vi "Process Image.vi"(4 "Path Angle":dbl, 6 "Camera Angle":dbl, 7 "Upper Threshold":dbl, 8 "Error In":errorcluster, 9 "FOV":dbl[](array[numeric]), 10 "Process Memory":T1, 11 "Acquired Image":T1) -> (0 "Error Out":errorcluster, 1 "Particle Locations":dbl[][](array[numeric]) format="%.2f", 2 "Processed Image":T1)   [LabVIEW 2017]
uses:
  <vilib>/vision/Image Controls.llb/IMAQ Image.ctl
  <vilib>/vision/NI_Vision_Development_Module.lvlib
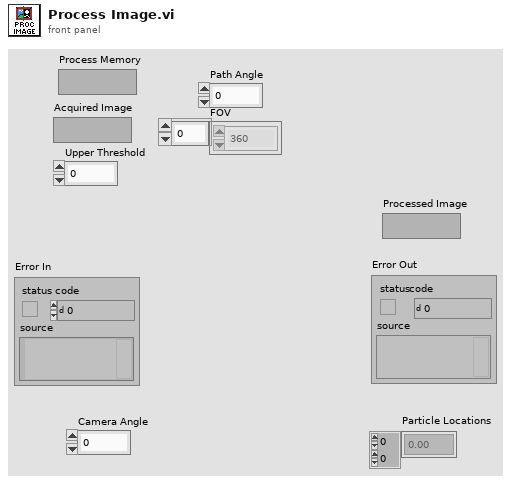
[diagram p1: front panel]
types:
  T1 = typedef "IMAQ Image.ctl" = refnum<image>
  T2 = typedef "IMAQ Circle" = cluster{"Center X":i32, "Center Y":i32, "Inner Radius":i32, "Outer Radius":i32, "Start Angle":dbl, "End Angle":dbl}
  T3 = typedef "Particle Parameters" = i32
  T4 = typedef "ROI Descriptor" = cluster{"Global Rectangle":i32[], "Contours":cluster{"ID":enum32{"External", "Internal"}, "Type":u32, "Coordinates":i32[]}[]}
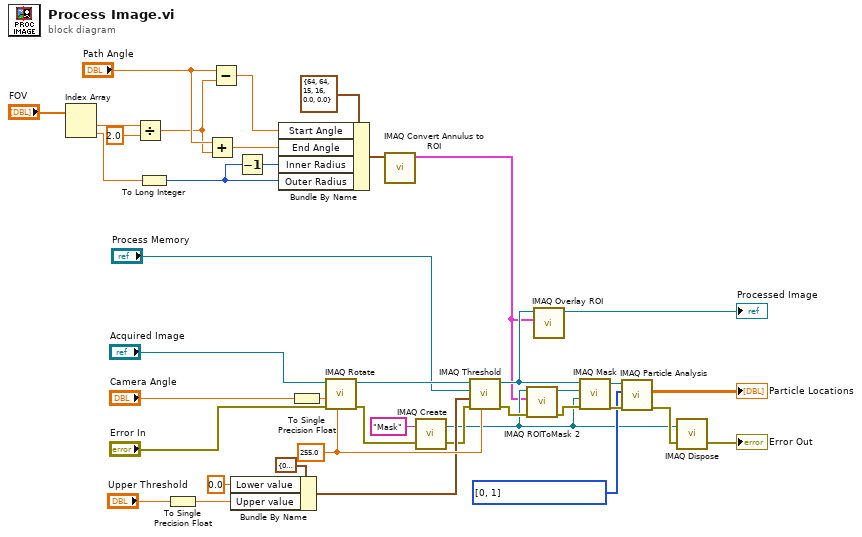
[diagram p0: block diagram]
diagram:
  w33 = T3[] [0, 1] items=["Center of Mass X", "Center of Mass Y", "First Pixel X", "First Pixel Y", "Bounding Rect Left", "Bounding Rect Top", "Bounding Rect Right", "Bounding Rect Bottom", "Max Feret Diameter Start X", "Max Feret Diameter Start Y", "Max Feret Diameter End X", "Max Feret Diameter End Y", "Max Horiz. Segment Length Left", "Max Horiz. Segment Length Right", "Max Horiz. Segment Length Row", "-", "Bounding Rect Width", "Bounding Rect Height", "Bounding Rect Diagonal", "Perimeter", "Convex Hull Perimeter", "Holes' Perimeter", "Max Feret Diameter", "Equivalent Ellipse Major Axis", "Equivalent Ellipse Minor Axis", "Equivalent Ellipse Minor Axis (Feret)", "Equivalent Rect Long Side", "Equivalent Rect Short Side", "Equivalent Rect Diagonal", "Equivalent Rect Short Side (Feret)", "Average Horiz. Segment Length", "Average Vert. Segment Length", "Hydraulic Radius", "Waddel Disk Diameter", "-", "Area", "Holes' Area", "Particle & Holes' Area", "Convex Hull Area", "Image Area", "-", "Number of Holes", "Number of Horiz. Segments", "Number of Vert. Segments", "-", "Orientation", "Max Feret Diameter Orientation", "-", "% Area/Image Area", "% Area/(Particle & Holes' Area)", "Ratio of Equivalent Ellipse Axes", "Ratio of Equivalent Rect Sides", "-", "Elongation Factor", "Compactness Factor", "Heywood Circularity Factor", "Type Factor", "-", "Sum X", "Sum Y", "Sum XX", "Sum XY", "Sum YY", "Sum XXX", "Sum XXY", "Sum XYY", "Sum YYY", "-", "Moment of Inertia XX", "Moment of Inertia XY", "Moment of Inertia YY", "Moment of Inertia XXX", "Moment of Inertia XXY", "Moment of Inertia XYY", "Moment of Inertia YYY", "Norm. Moment of Inertia XX", "Norm. Moment of Inertia XY", "Norm. Moment of Inertia YY", "Norm. Moment of Inertia XXX", "Norm. Moment of Inertia XXY", "Norm. Moment of Inertia XYY", "Norm. Moment of Inertia YYY", "Hu Moment 1", "Hu Moment 2", "Hu Moment 3", "Hu Moment 4", "Hu Moment 5", "Hu Moment 6", "Hu Moment 7"] ("Pixel Measurements")
  w40 = sgl 255.0 ("Replace Value")
  n1 = Index Array(array="FOV") -> (element #1=w4:dbl, element #2=w3:dbl)  [unwired: 2 in]
  n2 = Divide(x=w4, y=2.0) -> (x/y=w10:dbl)
  n3 = To Long Integer(number=w3) -> (32bit integer=w2:i32)
  n4 = To Single Precision Float(number="Upper Threshold") -> (single precision float=w6:sgl)
  n5 = Add(x="Path Angle", y=w10) -> (x+y=w9:dbl)
  n6 = Subtract(x="Path Angle", y=w10) -> (x-y=w8:dbl)
  n7 = Bundle By Name(cluster=cluster{"Lower value":sgl, "Upper value":sgl} {"Lower value"=0.0, "Upper value"=120.0} ("Threshold?"), "Lower value"=sgl 0.0, "Upper value"=w6) -> (w25:cluster{"Lower value":sgl, "Upper value":sgl})
  n8 = Decrement(x=w2) -> (x-1=w1:i32)
  n9 = Bundle By Name(cluster=T2 {"Center X"=64, "Center Y"=64, "Inner Radius"=15, "Outer Radius"=16, "Start Angle"=0.0, "End Angle"=0.0} ("Annulus"), "Start Angle"=w8, "End Angle"=w9, "Inner Radius"=w1, "Outer Radius"=w2) -> (w14:T2)
  n10 = To Single Precision Float(number="Camera Angle") -> (single precision float=w39:sgl)
  n11 = call "IMAQ Rotate"("Replace Value"=w40, "error in (no error)"="Error In", "Angle (degrees)"=w39, "Image Src"="Acquired Image") -> ("error out"=w20:errorcluster, "Image Dst Out"=w28:T1)  [unwired: 6 in]
  n12 = call "IMAQ Convert Annulus to ROI"("Annulus"=w14) -> ("ROI Descriptor"=w13:T4)  [unwired: 8 in, 1 out]
  n13 = call "IMAQ Create"("Image Name"="Mask", "error in (no error)"=w20) -> ("New Image"=w16:T1, "error out"=w19:errorcluster)  [unwired: 3 in]
  n14 = call "IMAQ Threshold"("Replace Value"=w40, "error in (no error)"=w19, "Range"=w25, "Image Dst"="Process Memory", "Image Src"=w28) -> ("error out"=w37:errorcluster, "Image Dst Out"=w23:T1)  [unwired: 5 in]
  n15 = call "IMAQ ROIToMask 2"("error in (no error)"=w37, "ROI Descriptor"=w13, "Image"=w16) -> ("error out"=w38:errorcluster, "Image Out"=w36:T1)  [unwired: 6 in, 1 out]
  n16 = call "IMAQ Overlay ROI"("ROI Descriptor"=w13, "Image"=w23) -> ("Image Out"=→"Processed Image":T1)  [unwired: 8 in, 1 out]
  n17 = call "IMAQ Mask"("error in (no error)"=w38, "Image Dst"=w16, "Image Mask"=w36, "Image Src"=w23) -> ("error out"=w35:errorcluster, "Image Dst Out"=w34:T1)  [unwired: 1 in]
  n18 = call "IMAQ Particle Analysis"("error in (no error)"=w35, "Pixel Measurements"=w33, "Image"=w34) -> ("error out"=w18:errorcluster, "Particle Measurements (Pixels)"=→"Particle Locations":dbl[][])  [unwired: 3 in, 4 out]
  n19 = call "IMAQ Dispose"("Image"=w16, "error in (no error)"=w18) -> ("error out"=→"Error Out":errorcluster)  [unwired: 4 in]
